vi "ReadConfigData.vi"(11 "ConfigData":path) -> (0 "Item MeasurementUnit":string[](array[string]), 1 "Item USL":string[](array[string]), 2 "Item LSL":string[](array[string]), 3 "ItemName":string[](array[string]))   [LabVIEW 2011]
uses:
  <vilib>/Utility/file.llb/Read From Spreadsheet File (string).vi
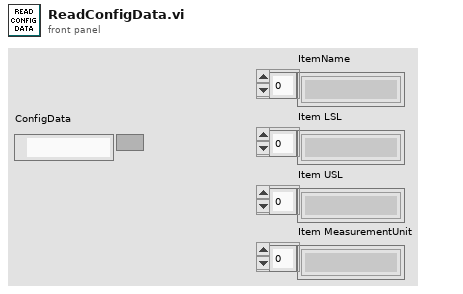
[diagram p1: front panel]
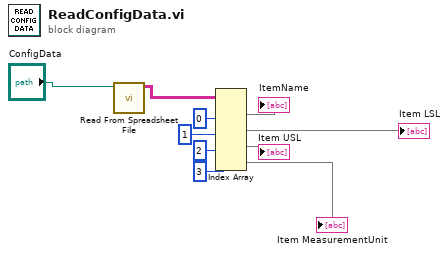
[diagram p0: block diagram]
diagram:
  n1 = call-poly <vilib>:"Read From Spreadsheet File.vi"("file path (dialog if empty)"="ConfigData") -> ("all rows"=w9:string[][])  [unwired: 6 in, 4 out]
  n2 = Index Array(array=w9, index (col) #1=0 ("禁用的索引 (列)"), index (col) #2=1 ("索引 (列)"), index (col) #3=2 ("索引 (列)"), index (col) #4=3 ("索引 (列)")) -> (element #1=→"ItemName":string[], element #2=→"Item LSL":string[], element #3=→"Item USL":string[], element #4=→"Item MeasurementUnit":string[])  [unwired: 4 in]
